vi "AutoChooseState.vi"(8 "error in (no error)":errorcluster, 9 "HotGoal?":bool, 10 "AutoMode":T2, 11 "AutoState":T1) -> (0 "error out":errorcluster, 3 "AutoState":T1)   [LabVIEW 2013]
uses:
  AutoStates.ctl
  AutoMode.ctl
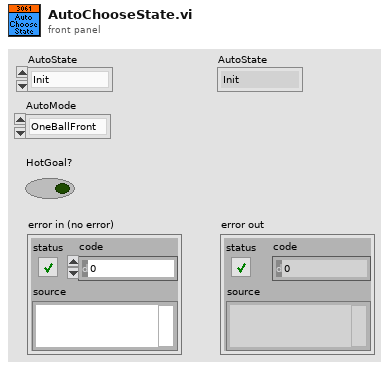
[diagram p1: front panel]
types:
  T1 = typedef "AutoStates.ctl" = enum16{"Init", "LowerArmCheckGoal", "DriveBack", "Collect", "StopCollect", "LiftArm", "RaiseServo", "Drive", "Wait", "ShootCollectorUp", "RaiseArm", "ShootCollectorDown", "Rotate1", "Rotate2", "Stop"}
  T2 = typedef "AutoMode.ctl" = enum16{"OneBallFront", "OneBallCollector", "TwoBallNormal", "TwoBallHot"}
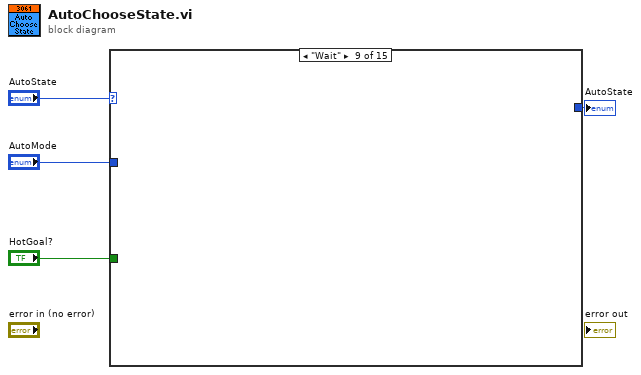
[diagram p0: block diagram]
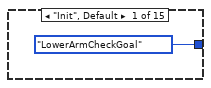
[diagram p2: hidden frame]
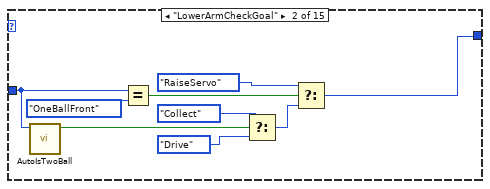
[diagram p3: hidden frame]
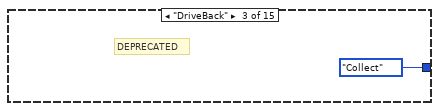
[diagram p4: hidden frame]
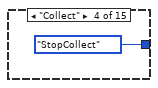
[diagram p5: hidden frame]
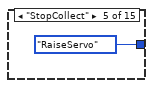
[diagram p6: hidden frame]
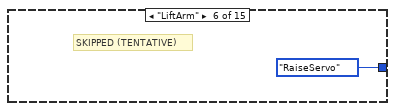
[diagram p7: hidden frame]
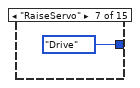
[diagram p8: hidden frame]
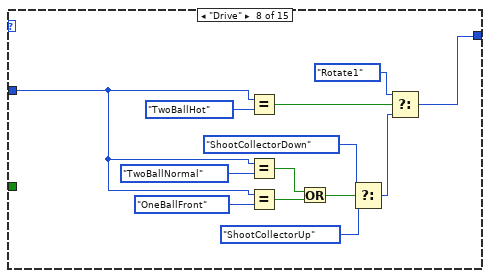
[diagram p9: hidden frame]
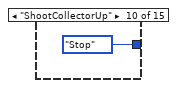
[diagram p10: hidden frame]
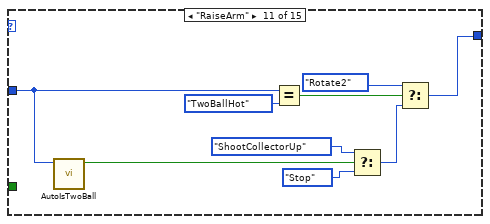
[diagram p11: hidden frame]
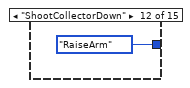
[diagram p12: hidden frame]
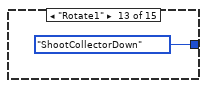
[diagram p13: hidden frame]
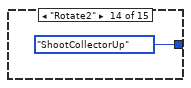
[diagram p14: hidden frame]
diagram:
  n1 = case shown="\"Wait\"" "AutoState" {
    selector: "AutoState" -> [_ _ _ _ _ _ _ _ _ _ _ _ _ _ w46]
    tunnel: "AutoMode" -> [_ w8 _ _ _ _ _ w20 _ _ w34 _ _ _ _]
    tunnel: "HotGoal?" -> [_ _ _ _ _ _ _ _ _ _ _ _ _ _ _]
    tunnel: [AutoStates."LowerArmCheckGoal" ("AutoState") w6 AutoStates."Collect" ("Enum") AutoStates."StopCollect" ("Enum") AutoStates."RaiseServo" ("Enum") AutoStates."RaiseServo" ("Enum") AutoStates."Drive" ("Enum") w22 _ AutoStates."Stop" ("f") w38 AutoStates."RaiseArm" ("Enum") AutoStates."ShootCollectorDown" ("Enum") AutoStates."ShootCollectorUp" ("Enum") w46] -> w1
    frame "Init", Default {
    }
    frame "LowerArmCheckGoal" {
      n2 = call "AutoIsTwoBall.vi"("AutoMode"=w8) -> ("IsTwoBall?"=w7:bool)  [unwired: 10 in]
      n3 = Equal?(x=w8, y=AutoMode."OneBallFront") -> (x = y?=w9:bool)
      n4 = Select(t=AutoStates."Collect" ("Enum"), s=w7, f=AutoStates."Drive" ("Enum")) -> (s? t:f=w11:T1)
      n5 = Select(t=AutoStates."RaiseServo" ("Enum"), s=w9, f=w11) -> (s? t:f=w6:T1)
    }
    frame "DriveBack" {
      # "DEPRECATED"
    }
    frame "Collect" {
    }
    frame "StopCollect" {
    }
    frame "LiftArm" {
      # "SKIPPED (TENTATIVE)"
    }
    frame "RaiseServo" {
    }
    frame "Drive" {
      n6 = Equal?(x=w20, y=AutoMode."TwoBallHot") -> (x = y?=w24:bool)
      n7 = Equal?(x=w20, y=AutoMode."TwoBallNormal") -> (x = y?=w31:bool)
      n8 = Equal?(x=w20, y=AutoMode."OneBallFront") -> (x = y?=w30:bool)
      n9 = Or(x=w31, y=w30) -> (x .or. y?=w26:bool)
      n10 = Select(t=AutoStates."ShootCollectorDown" ("Enum"), s=w26, f=AutoStates."ShootCollectorUp") -> (s? t:f=w25:T1)
      n11 = Select(t=AutoStates."Rotate1" ("Enum"), s=w24, f=w25) -> (s? t:f=w22:T1)
    }
    frame "Wait" {
    }
    frame "ShootCollectorUp" {
    }
    frame "RaiseArm" {
      n12 = call "AutoIsTwoBall.vi"("AutoMode"=w34) -> ("IsTwoBall?"=w37:bool)  [unwired: 10 in]
      n13 = Equal?(x=w34, y=AutoMode."TwoBallHot") -> (x = y?=w41:bool)
      n14 = Select(t=AutoStates."ShootCollectorUp" ("Enum"), s=w37, f=AutoStates."Stop" ("Enum")) -> (s? t:f=w39:T1)
      n15 = Select(t=AutoStates."Rotate2" ("Enum"), s=w41, f=w39) -> (s? t:f=w38:T1)
    }
    frame "ShootCollectorDown" {
    }
    frame "Rotate1" {
    }
    frame "Rotate2" {
    }
    frame "Stop" {
    }
  }
  "AutoState" <- w1
